vi "Digital Write Square Wave.vi"(7 "Duration (ms)":u32, 8 "Error In":errorcluster, 9 "Frequency (Hz)":u16, 10 "Channel":u8, 11 "LINX Resource":T1) -> (0 "Error Out":errorcluster, 3 "LINX Resource":T1)   [LabVIEW 2013, in "LVH-LINX.lvlib"]
doc: "Output a square wave with the specified frequency. myRIO uses PWM channels for this function while most other devices use a DO channel."
uses:
  <vilib>/LabVIEW Hacker/LINX/LVH-LINX.lvlib
  <vilib>/LabVIEW Hacker/LINX/Private/Type Defs/LINX Ref.ctl
  <vilib>/LabVIEW Hacker/LINX/Private/Type Defs/Platform.ctl
  <vilib>/LabVIEW Hacker/LINX/Private/Type Defs/Interface.ctl
  <vilib>/LabVIEW Hacker/LINX/Private/Device/Type Defs/LINX Device Config.ctl
  <vilib>/LabVIEW Hacker/LINX/Private/Device/Type Defs/TCP Config.ctl
  <vilib>/LabVIEW Hacker/LINX/Private/Type Defs/Device Family.ctl
  <vilib>/LabVIEW Hacker/LINX/Private/Type Defs/Peripheral.ctl
  <vilib>/LabVIEW Hacker/LINX/Private/Device/Device.lvlib
  <vilib>/LabVIEW Hacker/LINX/Private/myRIO/myRIO.lvlib
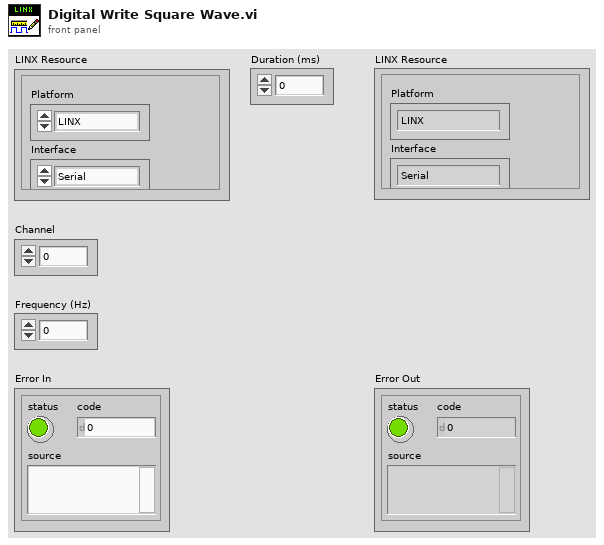
[diagram p1: front panel]
types:
  T1 = typedef "LVH-LINX.lvlib/LINX Ref.ctl" = cluster{"Platform":T2, "Interface":T3, "LINX Device Config":T4}
  T2 = typedef "LVH-LINX.lvlib/Platform.ctl" = enum16{"LINX", "myRIO"}
  T3 = typedef "LVH-LINX.lvlib/Interface.ctl" = enum16{"Serial", "TCP"}
  T4 = typedef "LVH-LINX.lvlib/Device.lvlib/LINX Device Config.ctl" = cluster{"Interface":T3, "COM Port":refnum<visa-resource-name>, "TCP Configuration":T5, "Device Family":T6, "Device ID":u8, "Device Name":string, "TCP Ref":refnum<k5>}
  T5 = typedef "LVH-LINX.lvlib/Device.lvlib/TCP Config.ctl" = cluster{"IP Address":string, "Port":u16}
  T6 = typedef "LVH-LINX.lvlib/Device Family.ctl" = enum8{"National Instruments", "Digilent", "Arduino"}
  T7 = typedef "LVH-LINX.lvlib/Peripheral.ctl" = enum8{"DI", "DO", "AI", "AO", "PWM", "QE", "UART", "I2C", "SPI", "CAN"}
  T8 = typedef "PWM.lvlib/PWM Reference.ctl" = cluster{"myRIO Reference":T9, "PWM Channels Enum":T13, "PWM Configuration":T14}
  T9 = typedef "myRIO Generic Hardware Reference.ctl" = cluster{"myRIO Model":T10, "myRIO Hardware Reference":T11}
  T10 = typedef "Hardware Version Enum.ctl" = enum16{"Unknown", "myRIO-1900", "myRIO-1950"}
  T11 = typedef "myRIO v1.0 Reference.ctl" = cluster{"Generic FPGA Reference":T12, "Allow multiple opens":bool}
  T12 = typedef "Generic FPGA Reference.ctl" = refnum<k20>
  T13 = typedef "PWM Channels Enum.ctl" = enum16{"Not Connected", "C/PWM0", "C/PWM1", "A/PWM0", "A/PWM1", "A/PWM2", "B/PWM0", "B/PWM1", "B/PWM2"}
  T14 = typedef "PWM.lvlib/PWM Configuration.ctl" = cluster{"Frequency":dbl, "Duty Cycle":dbl}
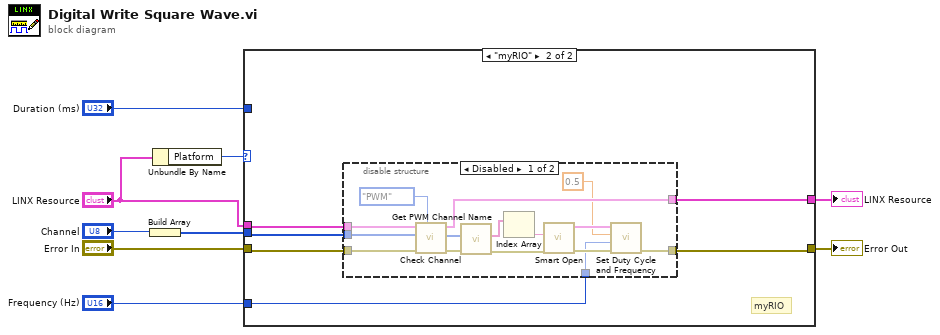
[diagram p0: block diagram]
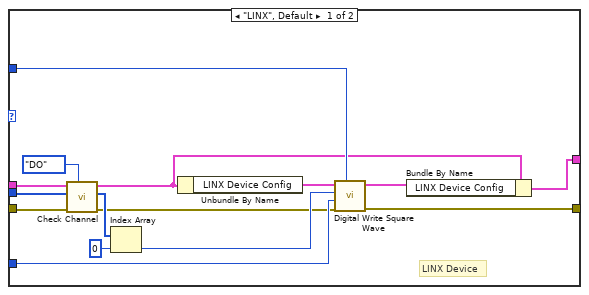
[diagram p2: hidden frame]
diagram:
  n1 = Build Array("Channel") -> (w2:u8[])
  n2 = Unbundle By Name("LINX Resource") -> ("Platform"=w9:T2)
  n3 = case shown="\"myRIO\"" w9 {
    tunnel: "Error In" -> [w16 w30]
    tunnel: "LINX Resource" -> [w13 w29]
    tunnel: [w20 w25] -> w8
    tunnel: [w24 w27] -> w7
    tunnel: w2 -> [w11 w28]
    tunnel: "Duration (ms)" -> [w17 _]
    tunnel: "Frequency (Hz)" -> [w18 w26]
    frame "LINX", Default {
      # "LINX Device"
      n4 = call <vilib>:"Check Channel.vi"("Peripheral"=Peripheral."DO", "Error In"=w16, "Channels"=w11, "LINX Resource"=w13) -> ("Error Out"=w14:errorcluster, "Channels"=w15:u8[], "LINX Resource"=w12:T1)  [unwired: 5 in]
      n5 = Index Array(array=w15, index=0) -> (element=w19:u8)
      n6 = Unbundle By Name(w12) -> ("LINX Device Config"=w22:T4)
      n7 = call <vilib>:"Digital Write Square Wave.vi"("Duration (ms)"=w17, "Error In"=w14, "Frequency"=w18, "DO Channel"=w19, "LINX Device Config"=w22) -> ("Error Out"=w20:errorcluster, "LINX Device Config"=w21:T4)  [unwired: 5 in]
      n8 = Bundle By Name(cluster=w12, "LINX Device Config"=w21) -> (w24:T1)
    }
    frame "myRIO" {
      # "myRIO"
      n9 = disable-structure shown="Disabled" {
        disable-tunnel: w30 -> [w43 _]
        disable-tunnel: w29 -> [w42 _]
        disable-tunnel: w28 -> [w40 _]
        disable-tunnel: [w39 _] -> w27
        disable-tunnel: w26 -> [w33 _]
        disable-tunnel: [w31 _] -> w25
        frame Disabled {
          n10 = call <vilib>:"Check Channel.vi"("Peripheral"=Peripheral."PWM", "Error In"=w43, "Channels"=w40, "LINX Resource"=w42) -> ("Error Out"=w44:errorcluster, "Channels"=w45:u8[], "LINX Resource"=w39:T1)  [unwired: 5 in]
          n11 = call <vilib>:"Get PWM Channel Name.vi"("Error In"=w44, "PWM Channel Nums"=w45) -> ("Error Out"=w36:errorcluster, "PWM Channels"=w35:string[])  [unwired: 8 in]
          n12 = Index Array(array=w35) -> (element=w34:string)  [unwired: 1 in]
          n13 = call <vilib>:"Smart Open.vi"("error in (no error)"=w36, "Channel Name"=w34) -> ("error out"=w37:errorcluster, "PWM Ref Out"=w38:T8)  [unwired: 8 in]
          n14 = call <vilib>:"Set Duty Cycle and Frequency.vi"("error in (no error)"=w37, "Frequency (Hz)"=w33, "Duty Cycle (0-1)"=0.5, "PWM Ref In"=w38) -> ("error out"=w31:errorcluster)  [unwired: 5 in, 1 out]
        }
        frame Enabled {
        }
      }
    }
  }
  "Error Out" <- w8
  "LINX Resource" <- w7
